vi "EvenSum&AverageMarcoGonzalez.vi"() -> ()   [LabVIEW 2012]
doc: "This VI will average and sum the first \"x\" even numbers. The user inputs \"x\" and displays both the sum and average."
panel:
  out "Average":dbl
  out "Sum":dbl
  in  "First":dbl
  # "Marco Gonzalez\nEA 3\n03 / 03 /2017"
  # "Even Numbers"
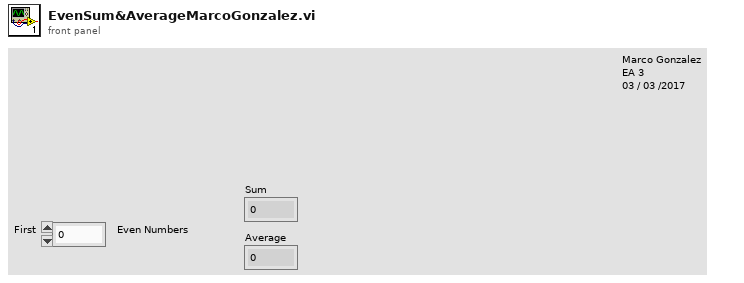
[diagram p1: front panel]
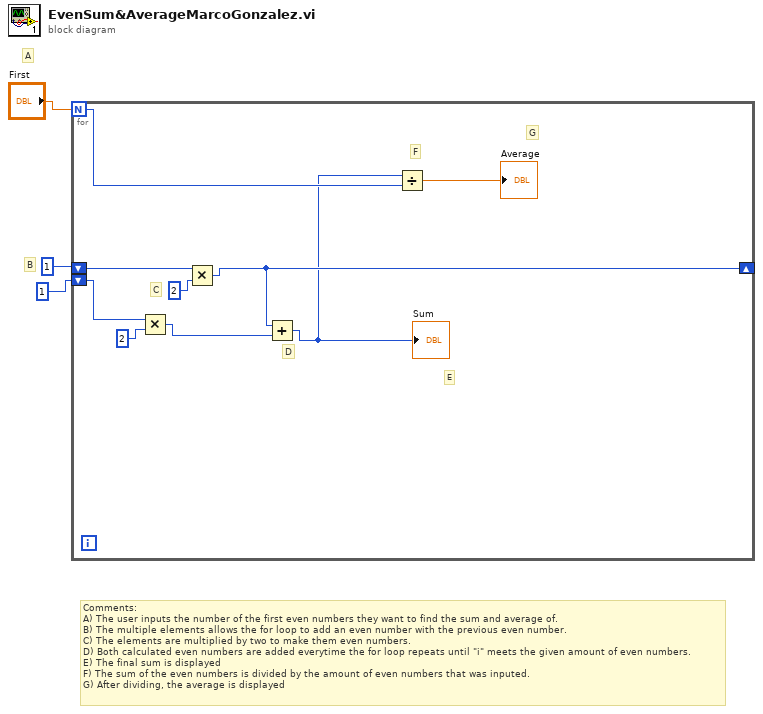
[diagram p0: block diagram]
diagram:
  # "B"
  # "A"
  # "Comments:\nA) The user inputs the number of the first even numbers they want to find the sum and average of.\nB) The multiple elements allows the for loop to add an even number with the previous even number.\nC) The elements are multiplied by two to make them even numbers.\nD) Both calculated even numbers are added everytime the for loop repeats until \"i\" meets the given amount of even numbers.\nE) The final sum is displayed\nF) The sum of the even numbers is divided by the amount of even numbers that was inputed.\nG) After dividing, the average is displayed"
  n1 = for {
    N: "First" -> [w8]
    shift-right: [w10] -> _
    shift-left: 1 -> [w11]
    shift-left: 1 -> [w5]
    # "G"
    # "F"
    # "E"
    # "D"
    # "C"
    n2 = Multiply(x=w5, y=2) -> (x*y=w4:i32)
    n3 = Multiply(x=w11, y=2) -> (x*y=w10:i32)
    n4 = Add(x=w10, y=w4) -> (x+y=w7:i32)
    "Sum" <- w7
    n5 = Divide(x=w7, y=w8) -> (x/y=→"Average":dbl)
  }
